vi "VALEW_Sensors_Current.vi"(0 "GEA2 Reference In":refnum<k24>, 1 "Lim_L_Current ADC Count":dbl[](array[numeric])=[0.0, 600.0, 1400.0, 1800.0, 2200.0, 3000.0, 3800.0], 3 "Lim_U_Current ADC Count":dbl[](array[numeric])=[200.0, 1000.0, 1800.0, 2200.0, 2600.0, 3400.0, 4200.0], 5 "GEA Inputs":T1={"Source"=228, "Destination"=35} {"Destination" format="%.0x"; "Source" format="%.0x"}, 7 "DAQmx Physical Channel":tag="9269_1/ao1", 9 "Array of Voltages":dbl[](array[numeric])=[0.0, 1.0, 2.0, 2.5, 3.0, 4.0, 5.0], 10 "Standalone?":bool, 11 "Error In":errorcluster, 12 "Lim_L_Current (A)":dbl[](array[numeric])=[14.0, 8.0, 2.0, 0.0, 2.0, 8.0, 14.0], 14 "Lim_U_Current (A)":dbl[](array[numeric])=[16.0, 10.0, 4.0, 1.0, 4.0, 10.0, 16.0]) -> (2 "Current ADC Count":dbl[](array[numeric]), 4 "GEA2 Reference Out":refnum<k24>, 6 "Pass/Fail?":bool, 8 "Report Text":string, 13 "Current (A)":dbl[](array[numeric]), 15 "Error Out":errorcluster)   [LabVIEW 2016, in "TL27.lvlib"]
uses:
  Projects/TL27.lvlib
  C:/Automation/DLLs/PC Dot Net/GeaCommunication.dll
  Common/LabVIEW GEA2 Toolkit/LabVIEW_GEA2_Toolkit.lvlibp/type defs/Source_Destination.ctl
  Common/LabVIEW GEA2 Toolkit/LabVIEW_GEA2_Toolkit.lvlibp/type defs/ERD Read Data In.ctl
  Common/LabVIEW GEA2 Toolkit/LabVIEW_GEA2_Toolkit.lvlibp/type defs/Data Type.ctl
  <vilib>/DAQmx/write.llb/DAQmx Write (Analog DBL 1Chan 1Samp).vi
  <vilib>/DAQmx/create/channels.llb/DAQmx Create Channel (AO-Voltage-Basic).vi
  <vilib>/DAQmx/miscellaneous.llb/DAQmx Fill In Error Info.vi
  Common/LabVIEW GEA2 Toolkit/LabVIEW_GEA2_Toolkit.lvlibp
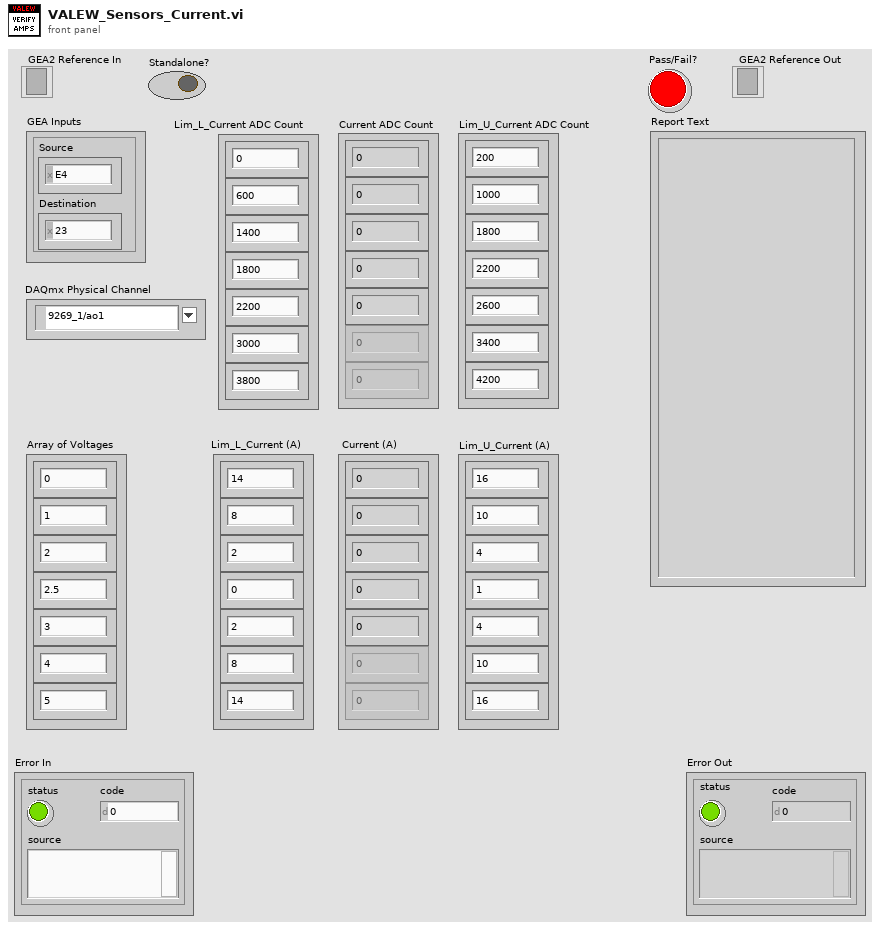
[diagram p1: front panel]
types:
  T1 = typedef "LabVIEW_GEA2_Toolkit.lvlibp/Source_Destination.ctl" = cluster{"Source":u8, "Destination":u8}
  T2 = typedef "LabVIEW_GEA2_Toolkit.lvlibp/ERD Read Data In.ctl" = cluster{"ERD Number":u16, "Data Type":T3}
  T3 = typedef "LabVIEW_GEA2_Toolkit.lvlibp/Data Type.ctl" = enum16{"string", "boolean", "uint8_t", "uint16_t", "uint32_t", "uint64_t", "int8_t", "int16_t", "int32_t", "int64_t"}
  T4 = typedef "LabVIEW_GEA2_Toolkit.lvlibp/ERD Read Data Out.ctl" = cluster{"ERD Number":u16, "Data":string}
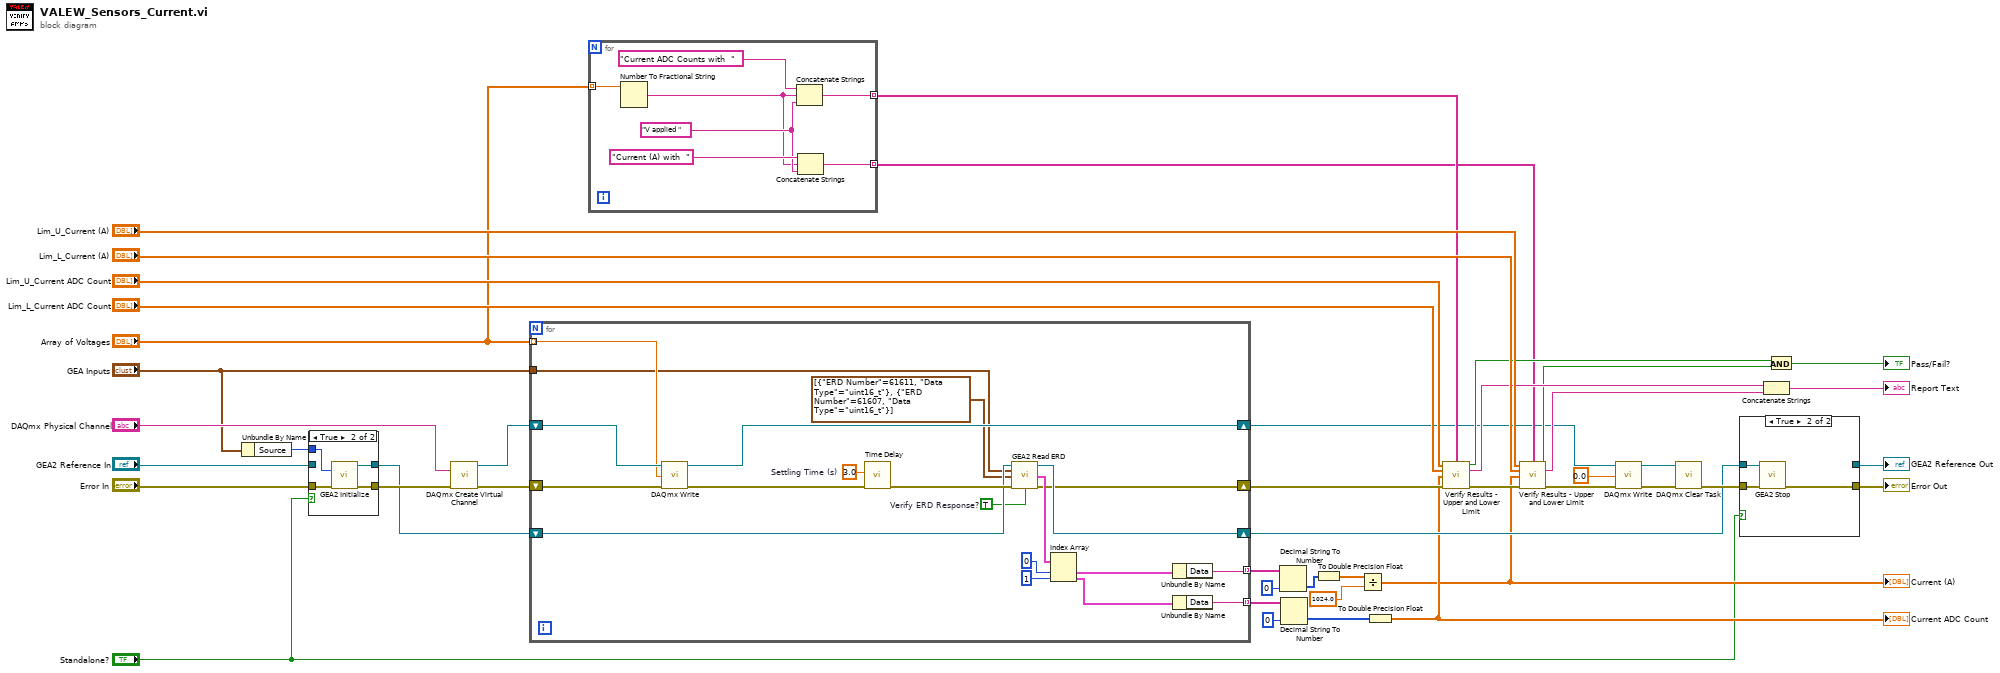
[diagram p0: block diagram]
diagram:
  n1 = Unbundle By Name("GEA Inputs") -> ("Source"=w33:u8)
  n2 = case shown="True" "Standalone?" {
    tunnel: "Error In" -> [w46 w50]
    tunnel: [w46 w49] -> w41
    tunnel: "GEA2 Reference In" -> [w45 _]
    tunnel: [w45 w48] -> w35
    tunnel: w33 -> [_ w47]
    frame False {
    }
    frame True {
      n3 = call "GEA2 Initialize.vi"("Source Address"=w47, "error in"=w50) -> ("GEA2 Reference Out"=w48:refnum<k24>, "error out"=w49:errorcluster)  [unwired: 11 in, 1 out]
    }
  }
  n4 = call-poly <vilib>:"DAQmx Create Virtual Channel.vi"("physical channels"="DAQmx Physical Channel", "error in"=w41) -> ("task out"=w38:refnum<k21>, "error out"=w40:errorcluster)  [unwired: 12 in]
  n5 = for {
    shift-right: [w52] -> w34
    shift-left: w35 -> [w64]
    shift-right: [w69] -> w2
    shift-left: w38 -> [w68]
    shift-right: [w51] -> w26
    shift-left: w40 -> [w70]
    tunnel: "GEA Inputs" -> [w57]
    tunnel: "Array of Voltages" -> [w63] mode=indexing
    tunnel: [w60] -> w31 mode=indexing
    tunnel: [w59] -> w28 mode=indexing
    w58 = TRUE  # Verify ERD Response?
    w67 = 3.0  # Settling Time (s)
    n6 = call-poly <vilib>:"DAQmx Write.vi"("task/channels in"=w68, "data"=w63, "error in"=w70) -> ("task out"=w69:refnum<k21>, "error out"=w65:errorcluster)  [unwired: 10 in, 1 out]
    n7 = call "Time Delay"("error in (no error)"=w65, "Delay Time (s)"=w67) -> ("error out"=w66:errorcluster)  [unwired: 9 in]
    n8 = call "GEA2 Read ERD.vi"("GEA2 Reference In"=w64, "GEA Inputs"=w57, "Read ERD List"=T2[] [{"ERD Number"=61611, "Data Type"=enum."uint16_t"}, {"ERD Number"=61607, "Data Type"=enum."uint16_t"}], "Error In"=w66, "Verify ERD Response?"=w58) -> ("GEA2 Reference Out"=w52:refnum<k24>, "ERD Data Out"=w62:T4[], "Error Out"=w51:errorcluster)  [unwired: 7 in, 1 out]
    n9 = Index Array(array=w62, index #1=0 ("index"), index #2=1 ("index")) -> (element #1=w55:T4, element #2=w54:T4)
    n10 = Unbundle By Name(w55) -> ("Data"=w59:string)
    n11 = Unbundle By Name(w54) -> ("Data"=w60:string)
  }
  n12 = for {
    tunnel: "Array of Voltages" -> [w77] mode=indexing
    tunnel: [w72] -> w7 mode=indexing
    tunnel: [w71] -> w8 mode=indexing
    w74 = "V applied "
    n13 = Number To Fractional String(number=w77) -> (F-format string=w73:string)  [unwired: 3 in]
    n14 = Concatenate Strings("Current ADC Counts with  ", w73, w74) -> (w71:string)
    n15 = Concatenate Strings("Current (A) with  ", w73, w74) -> (w72:string)
  }
  n16 = Decimal String To Number(string=w28, default (0L)=u32 0 ("default (0 I32)")) -> (number=w21:u32[])  [unwired: 1 in, 1 out]
  n17 = Decimal String To Number(string=w31, default (0L)=u16 0 ("default (0 I32)")) -> (number=w25:u16[])  [unwired: 1 in, 1 out]
  n18 = To Double Precision Float(number=w21) -> (double precision float=w22:dbl[])
  n19 = Divide(x=w22, y=1024.0) -> (x/y=w20:dbl[])
  "Current (A)" <- w20
  n20 = To Double Precision Float(number=w25) -> (double precision float=w24:dbl[])
  "Current ADC Count" <- w24
  n21 = call "Verify Results - Upper and Lower Limit.vi"("Upper Limits"="Lim_U_Current ADC Count", "Array of Names"=w8, "Lower Limits"="Lim_L_Current ADC Count", "Results"=w24, "Error In"=w26) -> ("Pass/Fail?"=w10:bool, "Report Text"=w14:string, "Error Out"=w27:errorcluster)  [unwired: 7 in, 1 out]
  n22 = call "Verify Results - Upper and Lower Limit.vi"("Upper Limits"="Lim_U_Current (A)", "Array of Names"=w7, "Lower Limits"="Lim_L_Current (A)", "Results"=w20, "Error In"=w27) -> ("Pass/Fail?"=w11:bool, "Report Text"=w15:string, "Error Out"=w5:errorcluster)  [unwired: 7 in, 1 out]
  n23 = call-poly <vilib>:"DAQmx Write.vi"("task/channels in"=w2, "data"=0.0, "error in"=w5) -> ("task out"=w3:refnum<k21>, "error out"=w4:errorcluster)  [unwired: 10 in, 1 out]
  n24 = call <vilib>:"DAQmx Clear Task.vi"("task in"=w3, "error in"=w4) -> ("error out"=w39:errorcluster)  [unwired: 13 in]
  n25 = case shown="True" "Standalone?" {
    tunnel: [w78 w82] -> w36
    tunnel: w34 -> [w79 w80]
    tunnel: [w79 _] -> w37
    tunnel: w39 -> [w78 w81]
    frame False {
    }
    frame True {
      n26 = call "GEA2 Stop.vi"("GEA2 Reference In"=w80, "Error In"=w81) -> ("Error Out"=w82:errorcluster)  [unwired: 13 in]
    }
  }
  "Error Out" <- w36
  "GEA2 Reference Out" <- w37
  n27 = Concatenate Strings(w14, w15) -> (→"Report Text":string)
  n28 = And(x=w10, y=w11) -> (x .and. y?=→"Pass/Fail?":bool)
